vi "New-Update Test.vi"(8 "error in (no error)":errorcluster, 10 "Test":refnum<class "TestManagerMsg.Test.lvclass">, 11 "Test Event Storage in":refnum<class "Test Event Storage.lvclass">) -> (0 "error out":errorcluster, 2 "updated?":bool, 3 "Test Event Storage out":refnum<class "Test Event Storage.lvclass">)   [LabVIEW 2020, in "Caraya.lvlib" / "Test Event Storage.lvclass"]
uses:
  Test Event Storage.lvclass
  Test Manager Message Test/TestManagerMsg.Test.lvclass
  C:/projects/caraya/src/classes/Test Manager Message/TestManagerMsg.lvclass
  Test Manager Message/TestManagerMsg.lvclass/TestManagerMsg.ctl
  Test Event Storage.lvclass/Test Event Storage.ctl
  test store -- cluster.ctl
  Test Manager Message/TestManagerMsg.lvclass
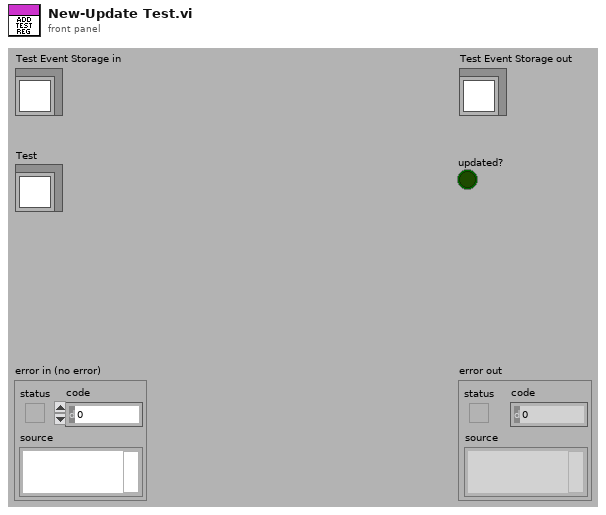
[diagram p1: front panel]
types:
  T1 = typedef "Caraya.lvlib/Test Event Storage.lvclass/test store -- cluster.ctl" = cluster{"Test":refnum<class "TestManagerMsg.Test.lvclass">, "Defined":bool, "Passed":bool, "properties":variant, "assert-ids":variant}
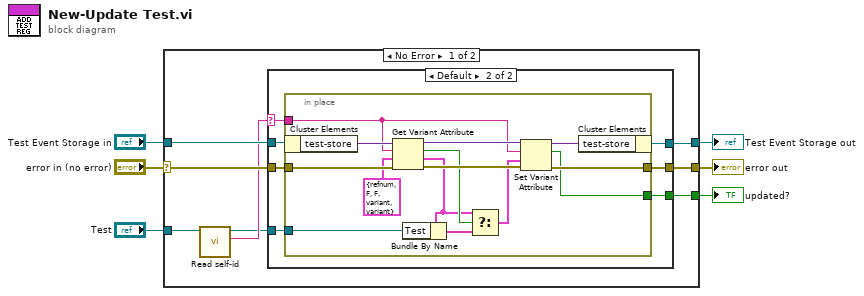
[diagram p0: block diagram]
diagram:
  n1 = case shown="No Error" "error in (no error)" {
    selector: "error in (no error)" -> [w10 w39]
    tunnel: [w14 w39] -> w5
    tunnel: [w13 w38] -> w3
    tunnel: "Test Event Storage in" -> [w11 w38]
    tunnel: [w12 _] -> w2
    tunnel: "Test" -> [w8 _]
    frame No Error {
      n2 = call "Read self-id.vi"("TestManagerMsg in"=w8) -> ("self-id"=w9:string, "TestManagerMsg out"=w7:refnum<class "TestManagerMsg.Test.lvclass">)  [unwired: 9 in]
      n3 = case shown="Default" w9 {
        selector: w9 -> [_ w19]
        tunnel: [w15 w23] -> w14
        tunnel: [w16 w22] -> w13
        tunnel: [_ w21] -> w12
        tunnel: w11 -> [w16 w18]
        tunnel: w10 -> [w15 w20]
        tunnel: w7 -> [_ w17]
        frame "" {
        }
        frame Default {
          n4 = in-place {
            in-place-border: w20 -> [w28]
            in-place-border: [w36] -> w23
            in-place-border: [w35] -> w21
            in-place-border: w17 -> [w26]
            in-place-border: w19 -> [w25]
            n5 = in-place-cluster #1(w18) -> ("test-store"=w29:variant)
            n6 = Get Variant Attribute(Variant=w29, name=w25, default value (empty Variant)=T1 {"Test"=refnum, "Defined"=FALSE, "Passed"=FALSE, "properties"=variant, "assert-ids"=variant} ("test-store"), error in=w28) -> (duplicate Variant=w34:variant, found=w32:bool, value=w30:T1, error out=w33:errorcluster)
            n7 = Bundle By Name(cluster=w30, "Test"=w26) -> (w24:T1)
            n8 = Select(t=w30, s=w32, f=w24) -> (s? t:f=w31:T1)
            n9 = Set Variant Attribute(Variant=w34, name=w25, value=w31, error in=w33) -> (Variant out=w37:variant, replaced=w35:bool, error out=w36:errorcluster)
            n10 = in-place-cluster #1("test-store"=w37) -> (w22:refnum<class "Test Event Storage.lvclass">)
          }
        }
      }
    }
    frame Error {
    }
  }
  "error out" <- w5
  "Test Event Storage out" <- w3
  "updated?" <- w2
